vi "Read Data Titles.vi"(8 "error in (no error)":errorcluster, 11 "LR-700 in":refnum<class "LR-700.lvclass">) -> (0 "error out":errorcluster, 2 "Data titles":string[](array[string])=["LR700_R (Ohm)", "LR700_X (Ohm)"], 3 "LR-700 out":refnum<class "LR-700.lvclass">)   [LabVIEW 2015, in "LR-700.lvclass"]
uses:
  LR-700.lvclass
  Instrument with scanner/Instrument with scanner Front Panel Data.ctl
  OO Devices/Device/Read Controls Snapshot.vi
  OO Devices/Device/Read Control Panel Loaded.vi
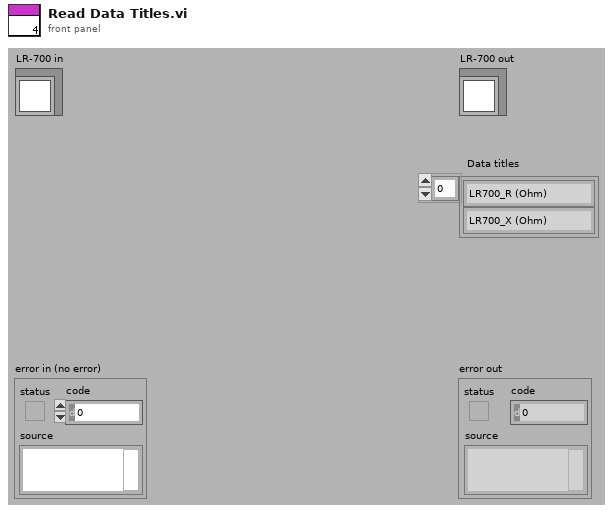
[diagram p1: front panel]
types:
  T1 = typedef "Instrument with scanner Front Panel Data.ctl" = cluster{"Channels to scan":i32[], "Scan settling, s":dbl}
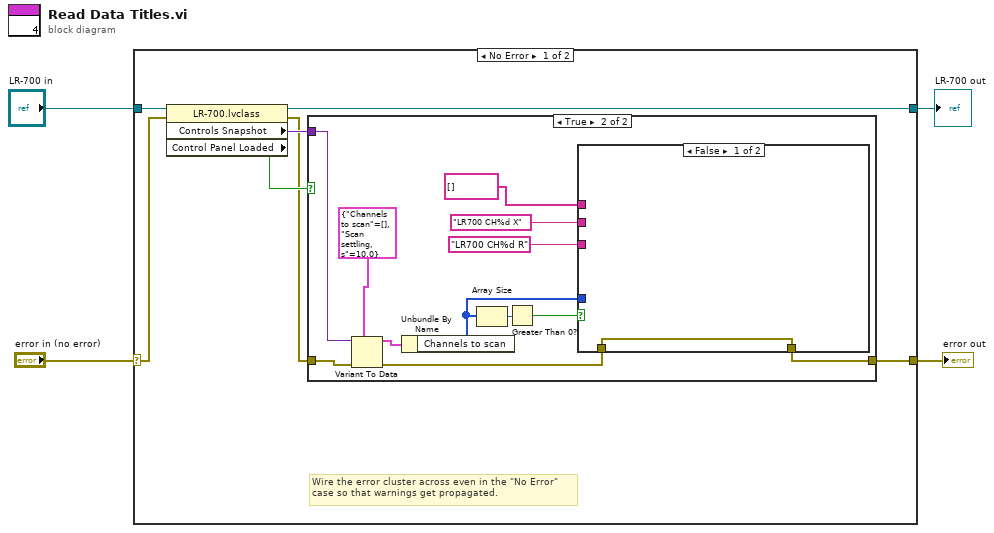
[diagram p0: block diagram]
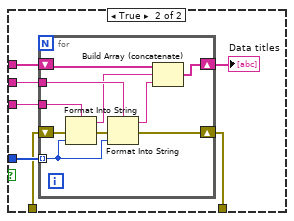
[diagram p3: hidden frame]
diagram:
  n1 = case shown="No Error" "error in (no error)" {
    selector: "error in (no error)" -> [w6 w44]
    tunnel: [w5 w44] -> w3
    tunnel: [w10 w43] -> w1
    tunnel: "LR-700 in" -> [w11 w43]
    frame No Error {
      # "Wire the error cluster across even in the \"No Error\"\ncase so that warnings get propagated."
      n2 = property class="LR-700.lvclass"(reference=w11, error in=w6) -> (reference out=w10:refnum<class "LR-700.lvclass">, error out=w7:errorcluster, "Controls Snapshot"=w8:variant, "Control Panel Loaded"=w9:bool)
      n3 = case shown="True" w9 {
        tunnel: w8 -> [_ w24]
        tunnel: w7 -> [w12 w23]
        tunnel: [w12 w13] -> w5
        frame False {
        }
        frame True {
          n4 = Variant To Data(error in=w23, type=T1 {"Channels to scan"=[], "Scan settling, s"=10.0} ("Data"), Variant=w24) -> (data=w21:T1, error out=w15:errorcluster)
          n5 = Unbundle By Name(w21) -> ("Channels to scan"=w18:i32[])
          n6 = Array Size(array=w18) -> (size(s)=w20:i32)
          n7 = Greater Than 0?(x=w20) -> (x > 0?=w19:bool)
          n8 = case shown="False" w19 {
            tunnel: w18 -> [_ w32]
            tunnel: "LR700 CH%d R" -> [_ w31]
            tunnel: "LR700 CH%d X" -> [_ w30]
            tunnel: w15 -> [w25 w29]
            tunnel: string[] [] -> [_ w28]
            tunnel: [w25 w26] -> w13
            frame False {
            }
            frame True {
              n9 = for {
                tunnel: w32 -> [w41] mode=indexing
                tunnel: w31 -> [w42]
                tunnel: w30 -> [w40]
                shift-right: [w38] -> w26
                shift-left: w29 -> [w39]
                shift-right: [w35] -> w27
                shift-left: w28 -> [w36]
                n10 = Format Into String(format string=w42, error in=w39, w41) -> (resulting string=w34:string, error out=w37:errorcluster)  [unwired: 1 in]
                n11 = Format Into String(format string=w40, error in=w37, w41) -> (resulting string=w33:string, error out=w38:errorcluster)  [unwired: 1 in]
                n12 = Build Array (concatenate)(w36, w34, w33) -> (w35:string[])
              }
              "Data titles" <- w27
            }
          }
        }
      }
    }
    frame Error {
    }
  }
  "error out" <- w3
  "LR-700 out" <- w1
